vi "Servo Lock.vi"(10 "Lock":bool, 11 "Enum":enum16{"Start", "Run", "End"}(ring)) -> ()   [LabVIEW 2012]
uses:
  TypeDefs/PWM Module 1.ctl
  <vilib>/Rock Robotics/SystemInterfaces/Typedef/FPGA_TypedefDigitalModule.ctl
  <vilib>/Rock Robotics/SystemInterfaces/DIO/FPGA_DIOPWMChannel.ctl
  <vilib>/Rock Robotics/SystemInterfaces/DIO/FPGA_DIORelayChannel.ctl
panel:
  in  "PWM Module (DIO A)":T1={"Module"=enum."Digital Module 1", "Shooter"=enum."PWM 1", "Right Drive"=enum."PWM 2", "Arm"=enum."PWM 3", "Left Drive"=enum."PWM 4", "Compress"=enum."PWM 5", "Arm Servo"=enum."PWM 6", "Unassigned"=enum."PWM 7", "Unassigned"=enum."PWM 8", "Unassigned"=enum."PWM 9", "Unassigned"=enum."PWM 10", "Loader"=enum."Relay 1", "Compressor"=enum."Relay 2", "Unassigned"=enum."Relay 3", "Unassigned"=enum."Relay 4", "Unassigned"=enum."Relay 5", "Unassigned"=enum."Relay 6", "Unassigned"=enum."Relay 7", "Unassigned "=enum."Relay 8"}
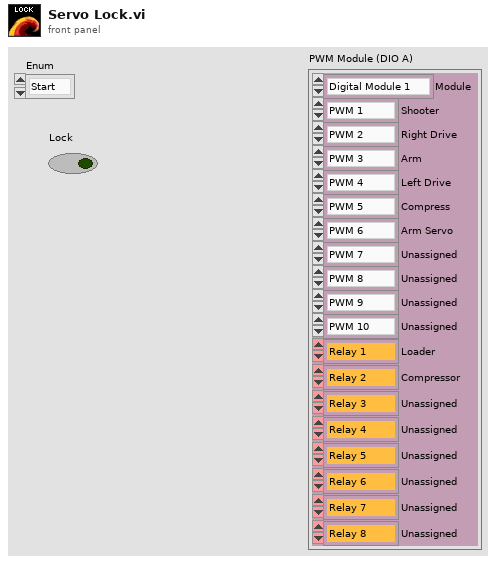
[diagram p1: front panel]
types:
  T1 = typedef "PWM Module 1.ctl" = cluster{"Module":T2, "Shooter":T3, "Right Drive":T3, "Arm":T3, "Left Drive":T3, "Compress":T3, "Arm Servo":T3, "Unassigned":T3, "Unassigned":T3, "Unassigned":T3, "Unassigned":T3, "Loader":T4, "Compressor":T4, "Unassigned":T4, "Unassigned":T4, "Unassigned":T4, "Unassigned":T4, "Unassigned":T4, "Unassigned ":T4}
  T2 = typedef "FPGA_TypedefDigitalModule.ctl" = enum16{"Digital Module 1", "Digital Module 2"}
  T3 = typedef "FPGA_DIOPWMChannel.ctl" = enum8{"PWM 1", "PWM 2", "PWM 3", "PWM 4", "PWM 5", "PWM 6", "PWM 7", "PWM 8", "PWM 9", "PWM 10", "Invalid"}
  T4 = typedef "FPGA_DIORelayChannel.ctl" = enum8{"Relay 1", "Relay 2", "Relay 3", "Relay 4", "Relay 5", "Relay 6", "Relay 7", "Relay 8", "Invalid"}
  T5 = typedef "WPI_ServoDeviceRef.ctl" = cluster{"DeviceStatus":errorcluster, "Digital Module":T2, "PWM Channel":T3, "DeadBand":T6}
  T6 = typedef "WPI_PWMDeadband.ctl" = cluster{"Name":string, "maxPositivePwm":i32, "minPositivePwm":i32, "centerPwm":i32, "maxNegativePwm":i32, "minNegativePwm":i32, "angularRange":u16}
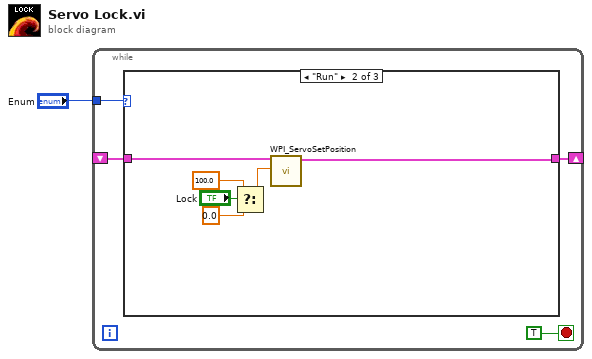
[diagram p0: block diagram]
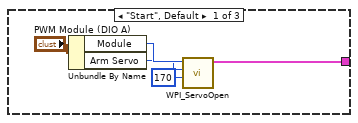
[diagram p2: hidden frame]
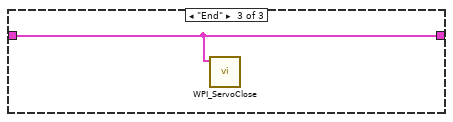
[diagram p3: hidden frame]
diagram:
  n1 = while {
    tunnel: "Enum" -> [w5]
    shift-right: [w4] -> _
    shift-left: _ -> [w3]
    stop <- TRUE stop-if-true
    n2 = case shown="\"Run\"" w5 {
      tunnel: [w6 w15 w17] -> w4
      tunnel: w3 -> [_ w16 w17]
      frame "Start", Default {
        n3 = Unbundle By Name("PWM Module (DIO A)") -> ("Module"=w9:T2, "Arm Servo"=w8:T3)
        n4 = call <vilib>:"WPI_ServoOpen.vi"("Angular Range"=u16 170, "PWM Channel"=w8, "Digital Module (Module 1)"=w9) -> ("ServoDeviceRef"=w6:T5)  [unwired: 7 in, 1 out]
      }
      frame "Run" {
        n5 = Select(t=100.0, s="Lock", f=0.0) -> (s? t:f=w11:dbl)
        n6 = call <vilib>:"WPI_ServoSetPosition.vi"("Position"=w11, "ServoDeviceRef"=w16) -> ("ServoDeviceRef"=w15:T5)  [unwired: 8 in, 1 out]
      }
      frame "End" {
        n7 = call <vilib>:"WPI_ServoClose.vi"("MotorControlDevRef"=w17) -> ()  [unwired: 10 in, 1 out]
      }
    }
  }
